vi "Open.vi"   [LabVIEW 2013, in "Mercury iXX.lvlib"]
doc: "Polymorphic open command can open a reference to the Mercury instrument or to a specific device within the instrument."
uses:
  <instrlib>/Mercury iXX/Mercury iXX.lvlib
  <instrlib>/Mercury iXX/Public/Libraries/System.lvlib
  <instrlib>/Mercury iXX/Public/Libraries/Magnet.lvlib
  <instrlib>/Mercury iXX/Public/Libraries/Heater.lvlib
  <instrlib>/Mercury iXX/Public/Libraries/Level Meter.lvlib
  <instrlib>/Mercury iXX/Public/Libraries/Temperature.lvlib
  <instrlib>/Mercury iXX/Public/Libraries/Auxiliary.lvlib
  <instrlib>/Mercury iXX/Public/Libraries/Pressure.lvlib
  <instrlib>/Mercury iXX/Public/Libraries/Flow.lvlib
  <instrlib>/Mercury iXX/Public/Libraries/Lambda.lvlib
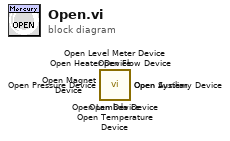
[diagram p0: block diagram]
diagram:
  n1 = call <instrlib>:"Open Lambda Device.vi"() -> ()  [unwired: 10 in, 2 out]
  n2 = call <instrlib>:"Open Flow Device.vi"() -> ()  [unwired: 10 in, 2 out]
  n3 = call <instrlib>:"Open Pressure Device.vi"() -> ()  [unwired: 10 in, 2 out]
  n4 = call <instrlib>:"Open Auxiliary Device.vi"() -> ()  [unwired: 10 in, 2 out]
  n5 = call <instrlib>:"Open Temperature Device.vi"() -> ()  [unwired: 10 in, 2 out]
  n6 = call <instrlib>:"Open Level Meter Device.vi"() -> ()  [unwired: 10 in, 2 out]
  n7 = call <instrlib>:"Open Heater Device.vi"() -> ()  [unwired: 10 in, 2 out]
  n8 = call <instrlib>:"Open Magnet Device.vi"() -> ()  [unwired: 10 in, 2 out]
  n9 = call <instrlib>:"Open Device.vi"() -> ()  [unwired: 10 in, 2 out]
  n10 = call <instrlib>:"Open System.vi"() -> ()  [unwired: 7 in, 5 out]
